vi "read data element message.vi"(8 "error in":errorcluster, 11 "data":variant) -> (0 "error out":errorcluster, 3 "data message":refnum<class "communicator message.lvclass">)   [LabVIEW 2015, in "connection maintainer.lvclass"]
uses:
  connection maintainer.lvclass
  message/communicator message.lvclass
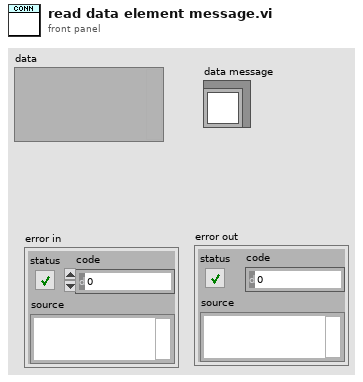
[diagram p1: front panel]
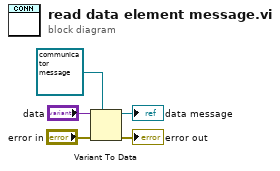
[diagram p0: block diagram]
diagram:
  n1 = Variant To Data(error in="error in", type=refnum<class "communicator message.lvclass"> refnum ("data message"), Variant="data") -> (data=→"data message":refnum<class "communicator message.lvclass">, error out=→"error out":errorcluster)
